vi "init_ccd_sbig.vi"(0 "Scan Directory":string="Peter_ferguson\\Tcal Labview\\test_scans\\", 1 "Exposure Time":dbl, 2 "Min nm":dbl, 3 "Max nm":dbl, 4 "Step size":dbl) -> (5 "Working Directory":path)   [LabVIEW 2018]
uses:
  <vilib>/Utility/sysdir.llb/System Directory Type.ctl
panel:
  out "Commands Sent":string
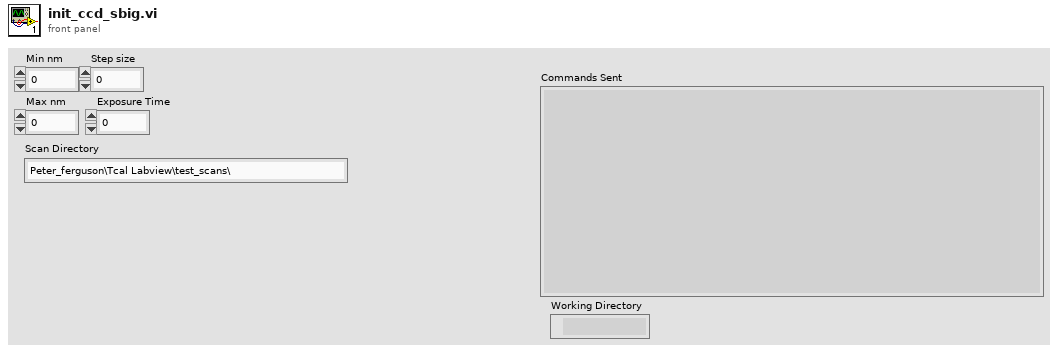
[diagram p1: front panel]
types:
  T1 = enum16{"open", "replace", "create", "open or create", "replace or create", "replace or create with confirmation"}
  T2 = typedef "System Directory Type.ctl" = i32
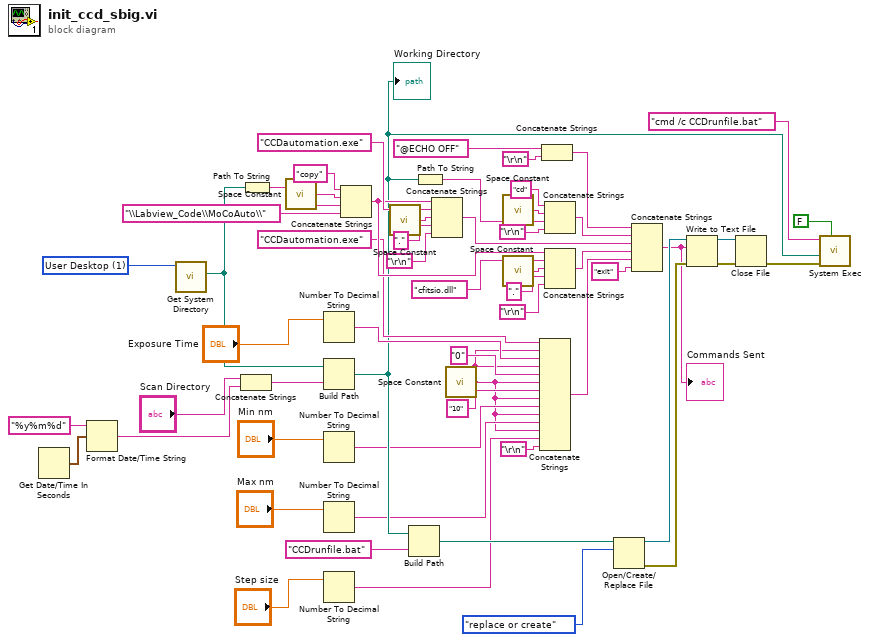
[diagram p0: block diagram]
diagram:
  w55 = T2 1 items=["User Home"=0, "User Desktop"=1, "User Documents"=2, "User Application Data"=3, "User Preferences"=4, "User Temporary"=5, "Public Documents"=6, "Public Application Data"=7, "Public Preferences"=8, "Public Cache"=13, "System Core Libraries"=9, "System Installed Libraries"=10, "Application Files"=11, "Boot Volume Root"=12] ("system directory type")
  n1 = Get Date/Time In Seconds() -> (seconds since 1Jan1904=w57:timestamp)
  n2 = Format Date/Time String(time format string (%c)="%y%m%d", seconds (now)=w57) -> (date/time string=w53:string)  [unwired: 1 in]
  n3 = call <vilib>:"Get System Directory.vi"("system directory type"=w55) -> ("system directory"=w51:path)  [unwired: 10 in]
  n4 = Concatenate Strings("Scan Directory", w53) -> (w52:string)
  n5 = Path To String(path=w51) -> (string=w42:string)
  n6 = call <vilib>:"Space Constant.vi"() -> ("String"=w43:string)
  n7 = Number To Decimal String(number="Exposure Time") -> (decimal integer string=w25:string)  [unwired: 1 in]
  n8 = Build Path(base path=w51, name or relative path=w52) -> (appended path=w12:path)
  "Working Directory" <- w12
  n9 = Number To Decimal String(number="Min nm") -> (decimal integer string=w5:string)  [unwired: 1 in]
  n10 = Number To Decimal String(number="Max nm") -> (decimal integer string=w4:string)  [unwired: 1 in]
  n11 = Number To Decimal String(number="Step size") -> (decimal integer string=w2:string)  [unwired: 1 in]
  n12 = Concatenate Strings("copy", w43, w42, "\\Labview_Code\\MoCoAuto\\" ("string")) -> (w33:string)
  n13 = call <vilib>:"Space Constant.vi"() -> ("String"=w37:string)
  n14 = Build Path(base path=w12, name or relative path="CCDrunfile.bat") -> (appended path=w19:path)
  n15 = Path To String(path=w12) -> (string=w46:string)
  n16 = Concatenate Strings(w33, "CCDautomation.exe" ("string"), w37, "." ("string"), "\r\n") -> (w34:string)
  n17 = call <vilib>:"Space Constant.vi"() -> ("String"=w3:string)
  n18 = call <vilib>:"Space Constant.vi"() -> ("String"=w47:string)
  n19 = call <vilib>:"Space Constant.vi"() -> ("String"=w31:string)
  n20 = Concatenate Strings("CCDautomation.exe" ("string"), w3, w25, w3, "0" ("string"), w3, "10" ("string"), w3, w5, w3, w4, w3, w2, "\r\n") -> (w8:string)
  n21 = Concatenate Strings("@ECHO OFF" ("string"), "\r\n") -> (w40:string)
  n22 = Concatenate Strings("cd" ("string"), w47, w46, "\r\n") -> (w39:string)
  n23 = Concatenate Strings(w33, "cfitsio.dll" ("string"), w31, "." ("string"), "\r\n") -> (w28:string)
  n24 = Open/Create/Replace File(file path (use dialog)=w19, operation (0:open)=T1."replace or create") -> (refnum out=w16:refnum<file>, error out=w15:errorcluster)  [unwired: 4 in, 1 out]
  n25 = Concatenate Strings(w40, w39, w34, w28, w8, "exit" ("string")) -> (w13:string)
  "Commands Sent" <- w13
  n26 = Write to Text File(file (use dialog)=w16, text=w13, error in=w15) -> (refnum out=w17:refnum<file>, error out=w14:errorcluster)  [unwired: 1 in, 1 out]
  n27 = Close File(refnum=w17, error in=w14) -> (error out=w9:errorcluster)  [unwired: 1 out]
  n28 = call <vilib>:"System Exec.vi"("wait until completion? (T)"=FALSE, "error in (no error)"=w9, "working directory"=w12, "command line"="cmd /c CCDrunfile.bat") -> ()  [unwired: 4 in, 4 out]
